vi "FTW-Test-JSON-Container.vi"() -> ()   [LabVIEW 2015]
panel:
  out "Match":bool
  out "error out":errorcluster
  in  "Pretty Print":bool=TRUE
  out "JSON String 2":string
  in  "JSON String":string="{\"a\":\"b\",\"c\":4}"
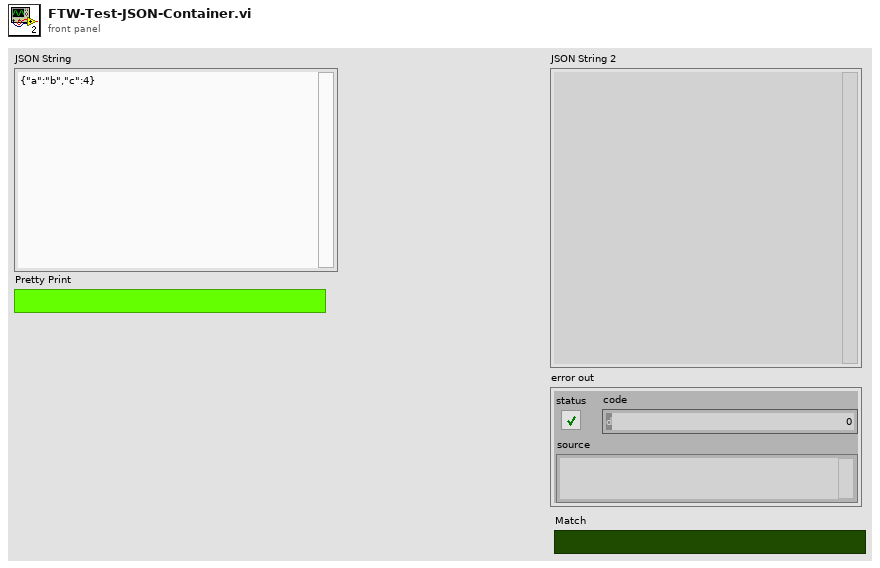
[diagram p1: front panel]
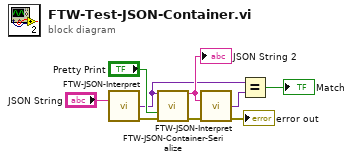
[diagram p0: block diagram]
diagram:
  n1 = call "FTW-JSON-Interpret.vi"("JSON String"="JSON String") -> ("Container"=w4:variant, "error out"=w9:errorcluster)  [unwired: 12 in, 1 out]
  n2 = call "FTW-JSON-Container-Serialize.vi"("Container"=w4, "Pretty Print"="Pretty Print", "error in"=w9) -> ("JSON String"=w6:string, "error out"=w3:errorcluster)  [unwired: 11 in]
  "JSON String 2" <- w6
  n3 = call "FTW-JSON-Interpret.vi"("JSON String"=w6, "error in"=w3) -> ("Container"=w5:variant, "error out"=→"error out":errorcluster)  [unwired: 11 in, 1 out]
  n4 = Equal?(x=w4, y=w5) -> (x = y?=→"Match":bool)
